vi "Test Data.vi"(8 "error in (no error)":errorcluster, 11 "Instrument.Lockin in":refnum<class "Instrument.Lockin.lvclass">) -> (0 "error out":errorcluster, 3 "Instrument.Lockin out":refnum<class "Instrument.Lockin.lvclass">)   [LabVIEW 2016]
uses:
  src/Instrument.Lockin/Instrument.Lockin.lvclass
  <vilib>/addons/_JKI Toolkits/Caraya/classes/Assert/Assert Not Error.vi
  <vilib>/addons/_JKI Toolkits/Caraya/classes/Assert/Assert False.vi
  <vilib>/addons/_JKI Toolkits/Caraya/classes/Test/Test.lvclass
  <vilib>/addons/_JKI Toolkits/Caraya/classes/Assert/Assert.lvclass
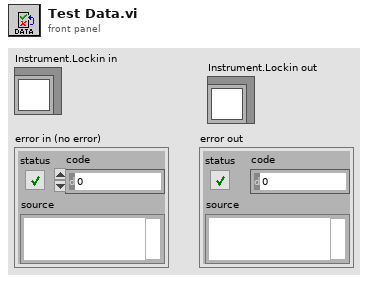
[diagram p1: front panel]
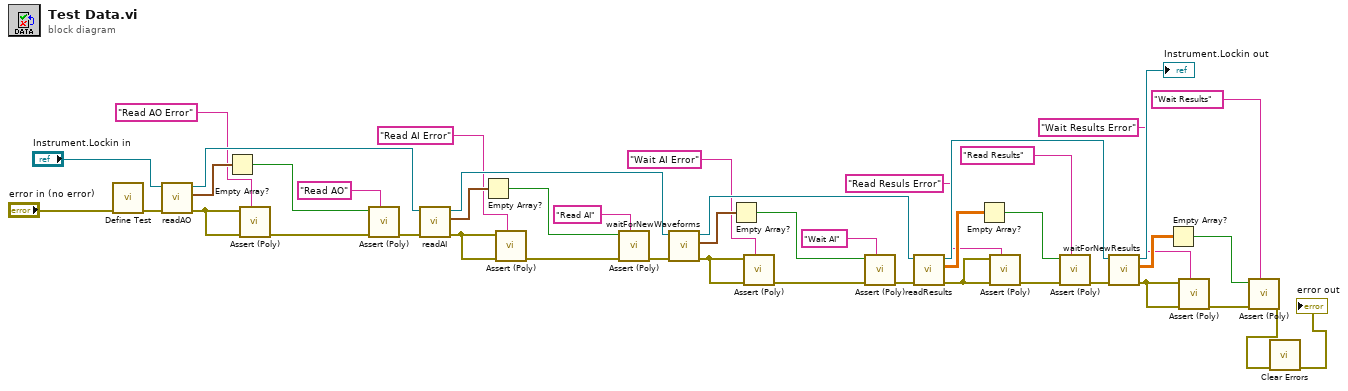
[diagram p0: block diagram]
diagram:
  n1 = call <vilib>:"Define Test.vi"("error in (no error)"="error in (no error)") -> ("error out"=w37:errorcluster)  [unwired: 10 in]
  n2 = call "readAO.vi"("error in (no error)"=w37, "Instrument.Lockin in"="Instrument.Lockin in") -> ("error out"=w36:errorcluster, "AO Waveforrm"=w31:waveform(dbl)[], "Instrument.Lockin out"=w41:refnum<class "Instrument.Lockin.lvclass">)  [unwired: 7 in]
  n3 = Empty Array?(array=w31) -> (empty?=w30:bool)
  n4 = call-poly <vilib>:"Assert (Poly).vi"("Label"="Read AO Error", "error in (no error)"=w36, "Not Error?"=w36) -> ("error out"=w29:errorcluster)  [unwired: 8 in]
  n5 = call-poly <vilib>:"Assert (Poly).vi"("Label"="Read AO", "error in (no error)"=w29, "False?"=w30) -> ("error out"=w22:errorcluster)  [unwired: 8 in]
  n6 = call "readAI.vi"("error in (no error)"=w22, "Instrument.Lockin in"=w41) -> ("error out"=w35:errorcluster, "AI Waveform"=w28:waveform(dbl)[], "Instrument.Lockin out"=w42:refnum<class "Instrument.Lockin.lvclass">)  [unwired: 7 in]
  n7 = Empty Array?(array=w28) -> (empty?=w27:bool)
  n8 = call-poly <vilib>:"Assert (Poly).vi"("Label"="Read AI Error", "error in (no error)"=w35, "Not Error?"=w35) -> ("error out"=w23:errorcluster)  [unwired: 8 in]
  n9 = call-poly <vilib>:"Assert (Poly).vi"("Label"="Read AI", "error in (no error)"=w23, "False?"=w27) -> ("error out"=w21:errorcluster)  [unwired: 8 in]
  n10 = call "waitForNewWaveforms.vi"("error in (no error)"=w21, "Instrument.Lockin in"=w42) -> ("error out"=w34:errorcluster, "Newest AI Waveform"=w26:waveform(dbl)[], "Instrument.Lockin out"=w43:refnum<class "Instrument.Lockin.lvclass">)  [unwired: 7 in]
  n11 = Empty Array?(array=w26) -> (empty?=w25:bool)
  n12 = call-poly <vilib>:"Assert (Poly).vi"("Label"="Wait AI Error", "error in (no error)"=w34, "Not Error?"=w34) -> ("error out"=w24:errorcluster)  [unwired: 8 in]
  n13 = call-poly <vilib>:"Assert (Poly).vi"("Label"="Wait AI", "error in (no error)"=w24, "False?"=w25) -> ("error out"=w20:errorcluster)  [unwired: 8 in]
  n14 = call "readResults.vi"("error in (no error)"=w20, "Instrument.Lockin in"=w43) -> ("error out"=w33:errorcluster, "Results"=w19:dbl[][], "Instrument.Lockin out"=w44:refnum<class "Instrument.Lockin.lvclass">)  [unwired: 6 in, 1 out]
  n15 = Empty Array?(array=w19) -> (empty?=w18:bool)
  n16 = call-poly <vilib>:"Assert (Poly).vi"("Label"="Read Resuls Error", "error in (no error)"=w33, "Not Error?"=w33) -> ("error out"=w17:errorcluster)  [unwired: 8 in]
  n17 = call-poly <vilib>:"Assert (Poly).vi"("Label"="Read Results", "error in (no error)"=w17, "False?"=w18) -> ("error out"=w13:errorcluster)  [unwired: 8 in]
  n18 = call "waitForNewResults.vi"("error in (no error)"=w13, "Instrument.Lockin in"=w44) -> ("error out"=w32:errorcluster, "Results"=w16:dbl[][], "Instrument.Lockin out"=→"Instrument.Lockin out":refnum<class "Instrument.Lockin.lvclass">)  [unwired: 7 in]
  n19 = Empty Array?(array=w16) -> (empty?=w15:bool)
  n20 = call-poly <vilib>:"Assert (Poly).vi"("Label"="Wait Results Error", "error in (no error)"=w32, "Not Error?"=w32) -> ("error out"=w14:errorcluster)  [unwired: 8 in]
  n21 = call-poly <vilib>:"Assert (Poly).vi"("Label"="Wait Results", "error in (no error)"=w14, "False?"=w15) -> ("error out"=w2:errorcluster)  [unwired: 8 in]
  n22 = call <vilib>:"Clear Errors.vi"("error in (no error)"=w2) -> ("error out"=→"error out":errorcluster)  [unwired: 5 in, 1 out]
